vi "Set Camera Mode Vision.vi"(1 "Set Camera Mode Message In":T1) -> (0 "Set Camera Mode Message Out":T1)   [LabVIEW 2016]
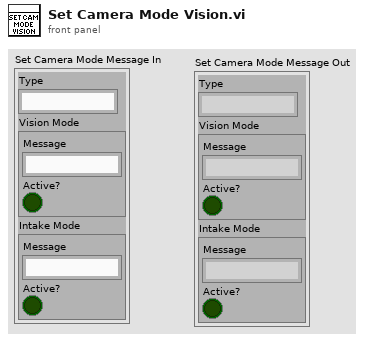
[diagram p1: front panel]
types:
  T1 = cluster{"Type":string, "Vision Mode":cluster{"Message":string, "Active?":bool}, "Intake Mode":cluster{"Message":string, "Active?":bool}}
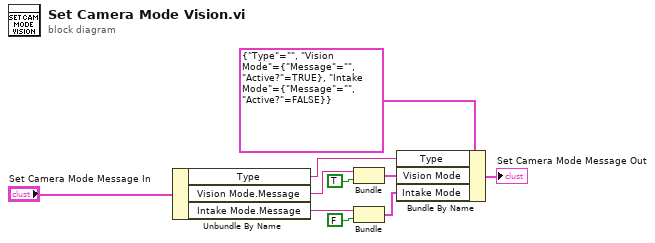
[diagram p0: block diagram]
diagram:
  n1 = Unbundle By Name("Set Camera Mode Message In") -> ("Type"=w7:string, "Vision Mode.Message"=w6:string, "Intake Mode.Message"=w3:string)
  n2 = Bundle("Message"=w6, "Active?"=TRUE) -> (w4:cluster{"Message":string, "Active?":bool})  [unwired: 1 in]
  n3 = Bundle("Message"=w3, "Active?"=FALSE) -> (w1:cluster{"Message":string, "Active?":bool})  [unwired: 1 in]
  n4 = Bundle By Name(cluster=T1 {"Type"="", "Vision Mode"={"Message"="", "Active?"=TRUE}, "Intake Mode"={"Message"="", "Active?"=FALSE}}, "Type"=w7, "Vision Mode"=w4, "Intake Mode"=w1) -> (→"Set Camera Mode Message Out":T1)
